vi "Publisher.vi"() -> ()   [LabVIEW 2019]
uses:
  Parameters.vi
panel:
  in  "stop":bool
  in  "Publisher":string
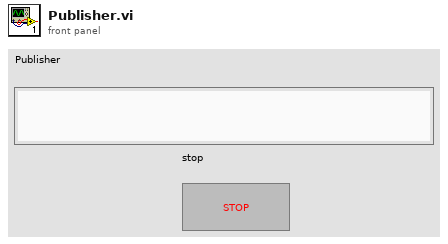
[diagram p1: front panel]
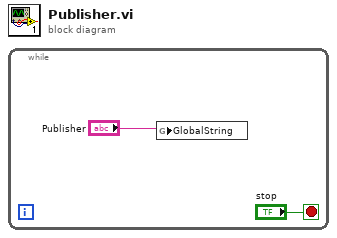
[diagram p0: block diagram]
diagram:
  n1 = while {
    stop <- "stop" stop-if-true
    n2 = global write "Parameters.vi" "GlobalString"("Publisher") -> ()
  }
